vi "nhv.vi"() -> ()   [LabVIEW 2011]
panel:
  out "Boolean 6":bool
  out "Boolean 5":bool
  out "Boolean 4":bool
  in  "Boolean 3":bool
  in  "Boolean 2":bool
  in  "Boolean":bool
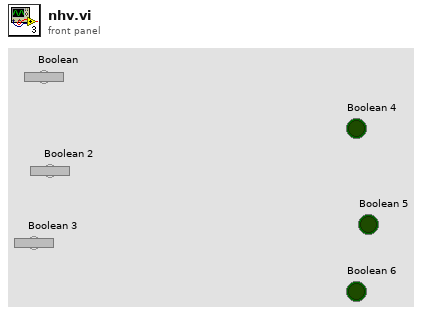
[diagram p1: front panel]
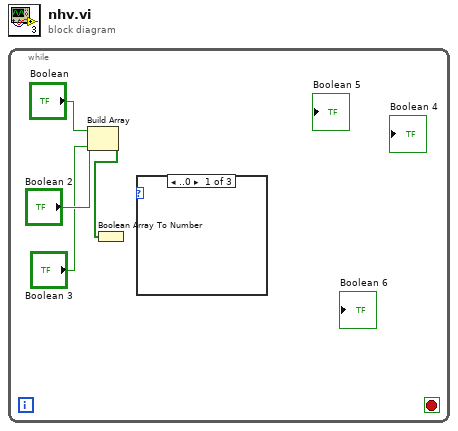
[diagram p0: block diagram]
diagram:
  n1 = while {
    stop <- _ stop-if-true
    n2 = Build Array("Boolean", "Boolean 2", "Boolean 3") -> (w1:bool[])
    n3 = Boolean Array To Number(Boolean array=w1) -> ()  [unwired: 1 out]
    n4 = case shown="..0" {
      selector: _ -> [_ _ _]
      frame ..0 {
      }
      frame 1 {
      }
      frame 2.. {
      }
    }
  }
